vi "UpdateInteger.vi"(8 "error in (no error)":errorcluster, 10 "Integer":i32, 11 "Model in":refnum<class "Model.lvclass">) -> (0 "error out":errorcluster, 3 "Model out":refnum<class "Model.lvclass">)   [LabVIEW 2020, in "Model.lvlib" / "Model.lvclass"]
uses:
  Model.lvclass
  Model.lvclass/Model.ctl
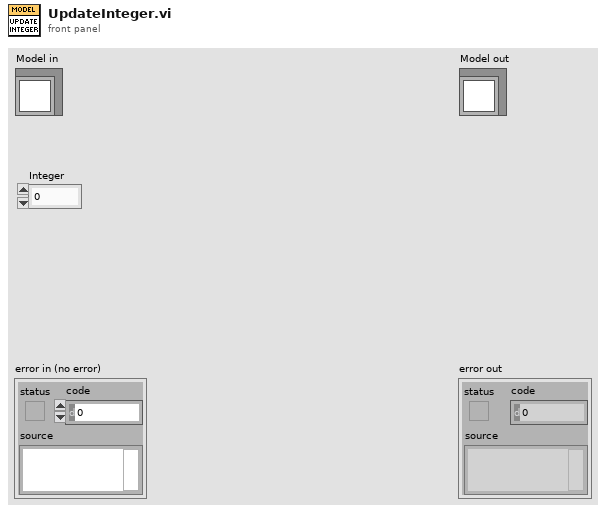
[diagram p1: front panel]
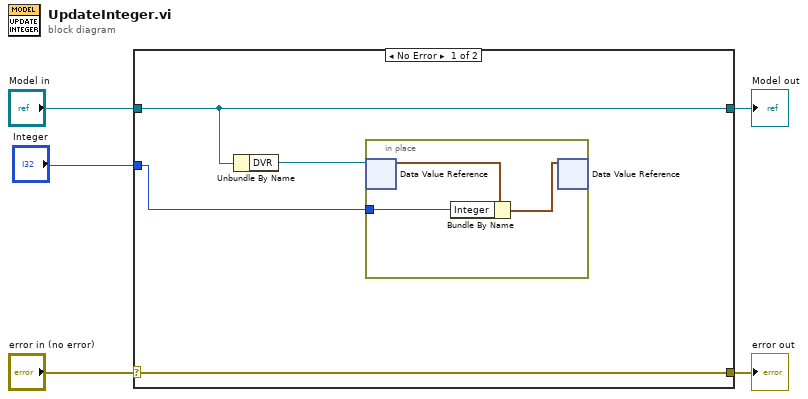
[diagram p0: block diagram]
diagram:
  n1 = case shown="No Error" "error in (no error)" {
    selector: "error in (no error)" -> [w9 w14]
    tunnel: [w9 w14] -> w4
    tunnel: [w8 w13] -> w2
    tunnel: "Model in" -> [w8 w13]
    tunnel: "Integer" -> [w6 _]
    frame No Error {
      n2 = Unbundle By Name(w8) -> ("DVR"=w7:refnum<data-value>)
      n3 = in-place {
        in-place-border: w6 -> [w10]
        n4 = in-place-dvr #1(w7) -> (w12:cluster{"Integer":i32})  [unwired: 1 out]
        n5 = Bundle By Name(cluster=w12, "Integer"=w10) -> (w11:cluster{"Integer":i32})
        n6 = in-place-dvr #1(w11) -> ()  [unwired: 2 out]
      }
    }
    frame Error {
    }
  }
  "error out" <- w4
  "Model out" <- w2
